vi "GetAll2TeamCombinations.vi"() -> ()   [LabVIEW 2018]
panel:
  out "Bye/DH Filler #":dbl
  out "# of Combinations":dbl
  out "Combinations":cluster{"Team 1":dbl, "Team 2":dbl}[](array[cluster])
  in  "# Teams":dbl
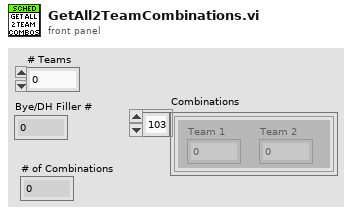
[diagram p1: front panel]
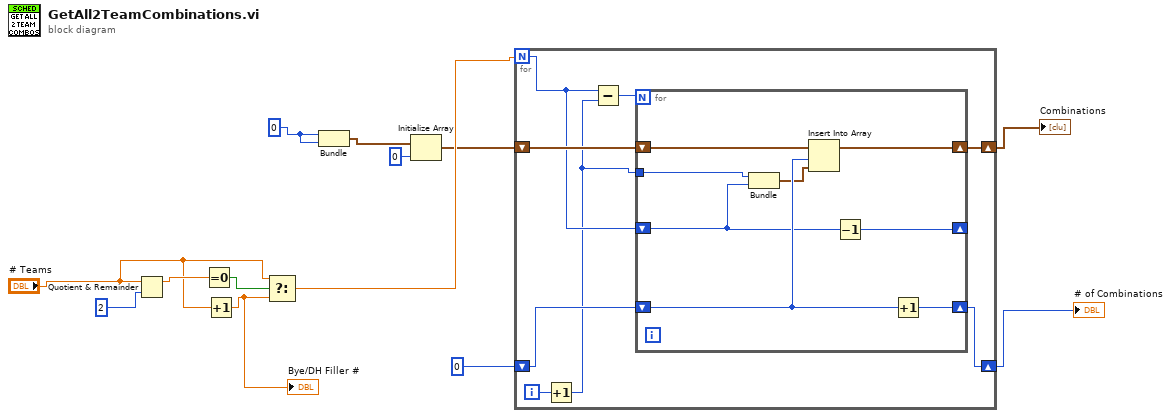
[diagram p0: block diagram]
diagram:
  w8 = 0
  n1 = Quotient & Remainder(x="# Teams", y=2) -> (x-y*floor(x/y)=w12:dbl)  [unwired: 1 out]
  n2 = Equal To 0?(x=w12) -> (x = 0?=w11:bool)
  n3 = Increment(x="# Teams") -> (x+1=w9:dbl)
  "Bye/DH Filler #" <- w9
  n4 = Select(t="# Teams", s=w11, f=w9) -> (s? t:f=w5:dbl)
  n5 = Bundle(w8, w8) -> (w7:cluster{i32, i32})  [unwired: 1 in]
  n6 = Initialize Array(w7, 0 ("dimension size")) -> (w4:cluster{i32, i32}[])
  n7 = for {
    N: w5 -> [w15]
    shift-right: [w20] -> w2
    shift-left: w4 -> [w21]
    shift-right: [w18] -> w1
    shift-left: 0 -> [w19]
    i -> [w16]
    n8 = Increment(x=w16) -> (x+1=w14:i32)
    n9 = Subtract(x=w15, y=w14) -> (x-y=w17:i32)
    n10 = for {
      N: w17 -> [_]
      shift-right: [w25] -> w20
      shift-left: w21 -> [w29]
      tunnel: w14 -> [w28]
      shift-right: [w26] -> w18
      shift-left: w19 -> [w27]
      shift-right: [w23] -> _
      shift-left: w15 -> [w22]
      n11 = Bundle(w28, w22) -> (w24:cluster{i32, i32})  [unwired: 1 in]
      n12 = Insert Into Array(array=w29, index=w27, new element=w24) -> (w25:cluster{i32, i32}[])
      n13 = Decrement(x=w22) -> (x-1=w23:i32)
      n14 = Increment(x=w27) -> (x+1=w26:i32)
    }
  }
  "Combinations" <- w2
  "# of Combinations" <- w1
